vi "Toggle IO Enable.vi"(8 "error in":errorcluster, 10 "IO_EN":bool, 11 "DIG_IO in":refnum<class "DIG_IO.lvclass">) -> (0 "error out":errorcluster, 3 "DIG_IO out":refnum<class "DIG_IO.lvclass">)   [LabVIEW 2019, in "DIG_IO.lvlib" / "DIG_IO.lvclass"]
doc: "This VI Is provided in support of the SLSC Chassis operation where the outputs can be enabled/disabled as a protection for flight hardware."
uses:
  Library/DIG_IO.lvclass
  C:/Users/Public/Documents/Development/builds/Instruments/Instruments.lvlibp/Library/Instruments.lvclass
  Library/DIG_IO.lvclass/DIG_IO.ctl
  builds/Instruments/Instruments.lvlibp/Private/Polymorphic/Special/Event from Boolean.vi
  builds/Instruments/Instruments.lvlibp/Accessors/Command with Logging.vi
  builds/Instruments/Instruments.lvlibp/Library/Instruments.lvclass
  builds/Instruments/Instruments.lvlibp
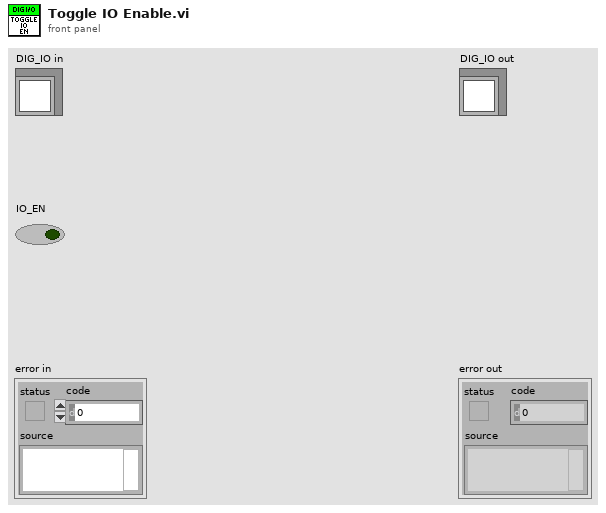
[diagram p1: front panel]
types:
  T1 = cluster{"Timestamp":timestamp, "Description":string, "Data":string}
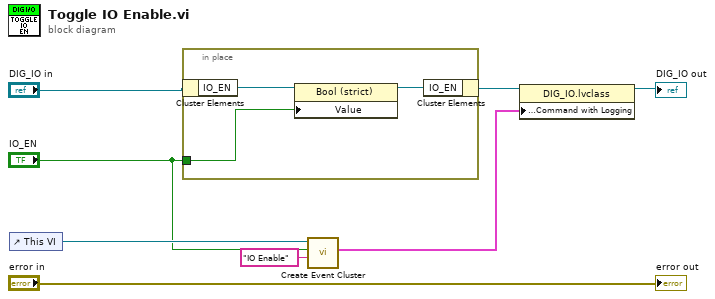
[diagram p0: block diagram]
diagram:
  n1 = control-ref of="This VI"() -> (w4:refnum<vi>)
  n2 = in-place {
    in-place-border: "IO_EN" -> [w9]
    n3 = in-place-cluster #1("DIG_IO in") -> ("IO_EN"=w11:refnum<vi>)
    n4 = property class="Bool (strict)"(reference=w11, "Value"=w9) -> (reference out=w10:refnum<vi>)  [unwired: 1 in, 1 out]
    n5 = in-place-cluster #1("IO_EN"=w10) -> (w7:refnum<class "DIG_IO.lvclass">)
  }
  n6 = call-poly "Create Event Cluster.vi"("Name"="IO Enable", "Value"="IO_EN", "VI Refnum"=w4) -> ("Event Data"=w1:T1)  [unwired: 8 in]
  n7 = property class="DIG_IO.lvclass"(reference=w7, "Accessors:Logging:Command with Logging"=w1) -> (reference out=→"DIG_IO out":refnum<class "DIG_IO.lvclass">)  [unwired: 1 in, 1 out]
  "error out" <- "error in"
